vi "S2C_CMD_FindRtns.vi"(8 "Error In":errorcluster, 11 "Command":string) -> (0 "Error Out":errorcluster, 3 "AllRtns":string[](array[string]))   [LabVIEW 2015]
doc: "Finds the return values associated with a command."
uses:
  S2C_CMD_Globals.vi
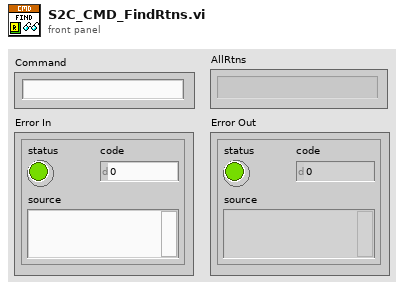
[diagram p1: front panel]
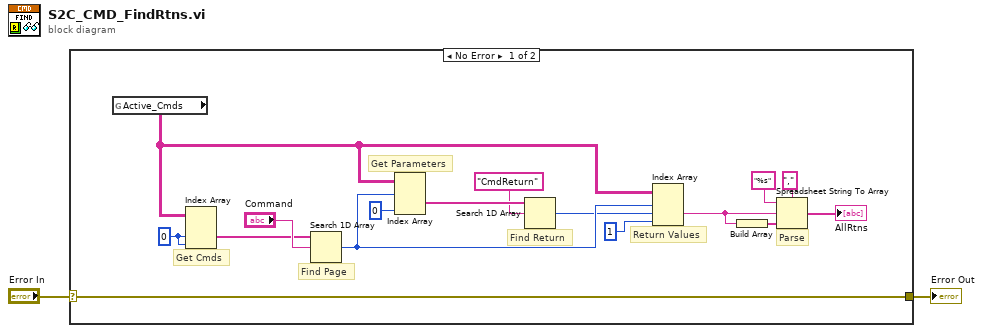
[diagram p0: block diagram]
diagram:
  n1 = case shown="No Error" "Error In" {
    selector: "Error In" -> [w15 w19]
    tunnel: [w15 w19] -> w1
    frame No Error {
      w18 = 0 ("disabled index (row)")
      # "Parse"
      # "Return Values"
      # "Find Return"
      # "Get Parameters"
      # "Find Page"
      # "Get Cmds"
      n2 = global read "S2C_CMD_Globals.vi" "Active_Cmds"() -> (w11:string[][][])
      n3 = Index Array(array=w11, index (dim 1)=w18, index (dim 2)=w18) -> (element=w14:string[])  [unwired: 1 in]
      n4 = Search 1D Array(1D array=w14, element="Command") -> (index of element=w10:i32)  [unwired: 1 in]
      n5 = Index Array(array=w11, index (dim 0)=w10, index (dim 2)=0 ("disabled index (col)")) -> (element=w13:string[])  [unwired: 1 in]
      n6 = Search 1D Array(1D array=w13, element="CmdReturn") -> (index of element=w9:i32)  [unwired: 1 in]
      n7 = Index Array(array=w11, index (dim 0)=w10, index (dim 1)=w9, index (dim 2)=1 ("disabled index (col)")) -> (element=w5:string)
      n8 = Build Array(w5) -> (w4:string[])
      n9 = Spreadsheet String To Array(delimiter (Tab)=",", format string="%s", spreadsheet string=w5, array type (2D Dbl)=w4) -> (array=→"AllRtns":string[])
    }
    frame Error {
    }
  }
  "Error Out" <- w1
